vi "RT Driver VI.vi"(6 "Device Clock":string, 9 "Device Inputs FIFO":refnum<k33>, 10 "Device Outputs FIFO":refnum<k33>, 11 "Device Reference":T1 format="%.0x") -> ()   [LabVIEW 2019, in "Reset Hardware Engine.lvlib"]
uses:
  Reset Hardware Engine.lvlib
  <vilib>/NI VeriStand/Custom Device API/Custom Device Channel Type.ctl
  <vilib>/NI VeriStand/Custom Device API/Custom Device API.lvlib
  <vilib>/NI VeriStand/Custom Device Tools/Custom Device Utility Library/Custom Device Utility Library.lvlib
  <vilib>/NI VeriStand/Custom Device API/Message Response (String).ctl
  <vilib>/NI VeriStand/Custom Device API/Message Response (Byte Array).ctl
  Shared/Compiled.Settings.ctl
  Shared/Reset Hardware Shared.lvlib
  Shared/Constants.vi
  <vilib>/NI VeriStand/Custom Device API/Get Item Property (Variant).vi
  <vilib>/NI VeriStand/Custom Device API/Custom Device Item Ref.ctl
panel:
  in  "Initialization Status Notifier":refnum<notifier>
  in  "Status Notifier":refnum<notifier>
  # "Custom Device Template\nv1.0"
  # "Use this template as a starting point for creating a custom device code module. The input controls shown here are specially named controls that the system will use to provide the device loop with data. The controls are not required for the device loop to run. For instance, if the device doesn't produce any output data, then you don't need the Device Outputs FIFO control. If you do use these controls, however, they need to have these exact names to be functional."
  # "The optional status notifier element is used to notify the RT engine of the last state of the custom device, and to indicate the device has completed execution. If this control is not used, a default No Error value is returned to the system when the device finishes execution.\n\nNote: This error state is not checked until the system shuts down. Use an output status channel to send more immediate status values to the system."
  # "This optional input can be used to send the VeriStand Engine the final status of the custom device initalization process. If this control exists on the custom device front panel, the VeriStand Engine will wait for a status update before starting up. If the custom device reports an error, that will abort the execution of the current configuration in the VeriStand Engine.\n\nThis control can be deleted if the custom device does not need to send the initialization status update."
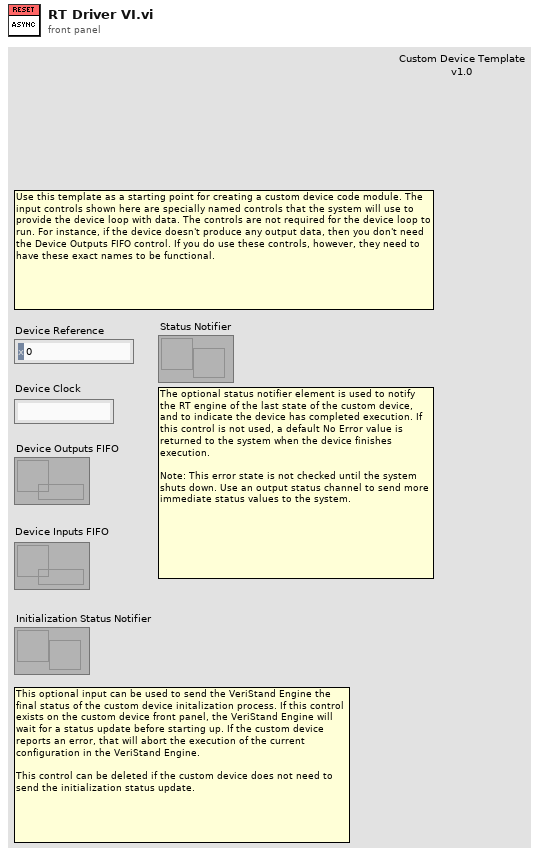
[diagram p1: front panel]
types:
  T1 = typedef "Custom Device API.lvlib/Custom Device Item Ref.ctl" = u64
  T2 = typedef "Reset Hardware Shared.lvlib/Compiled.Settings.ctl" = cluster{"Name":string, "Reset DAQmx AO":bool, "Reset XNET":bool}
  T3 = typedef "Custom Device API.lvlib/Custom Device Channel Type.ctl" = enum16{"Input", "Output"}
  T4 = typedef "Custom Device API.lvlib/Custom Device Engine Event Ref.ctl" = refnum<event-registration>
  T5 = typedef "Custom Device API.lvlib/Message Response (String).ctl" = cluster{"Response":string, "Error":errorcluster}
  T6 = typedef "Custom Device API.lvlib/Message Response (Byte Array).ctl" = cluster{"Response":u8[], "Error":errorcluster}
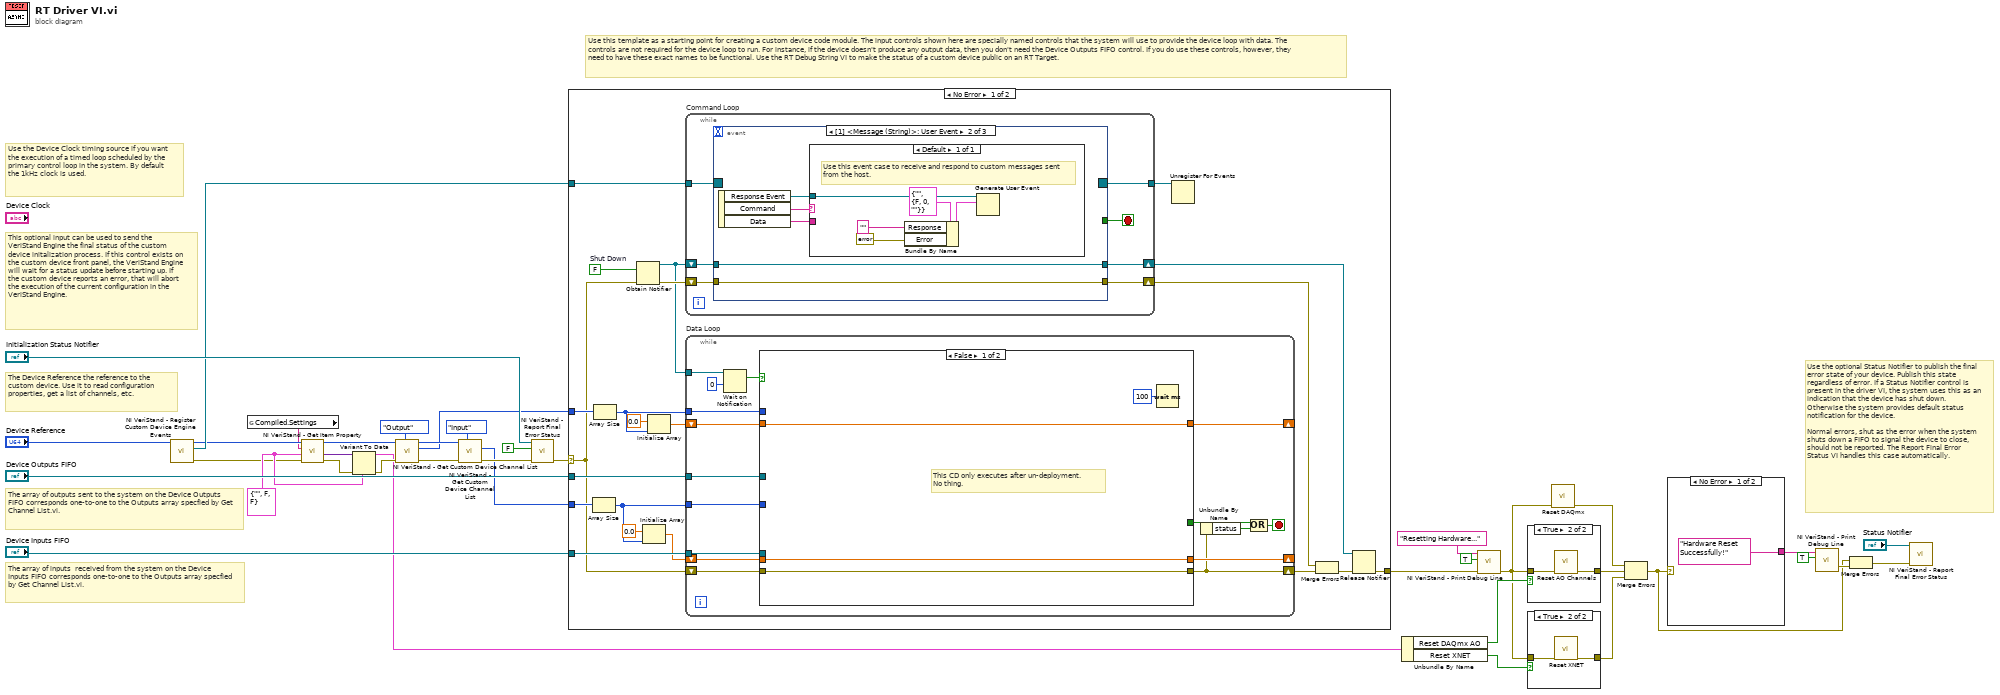
[diagram p0: block diagram]
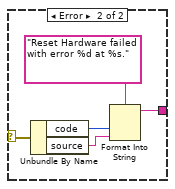
[diagram p4: hidden frame]
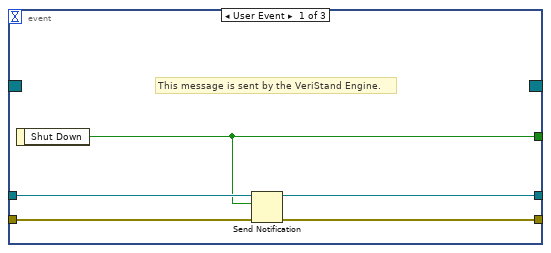
[diagram p5: hidden frame]
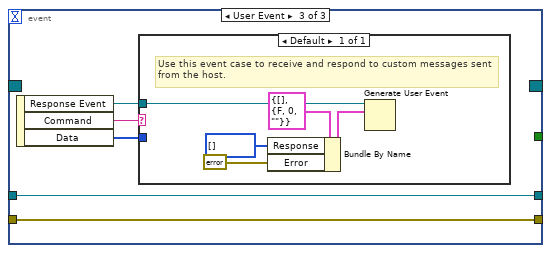
[diagram p6: hidden frame]
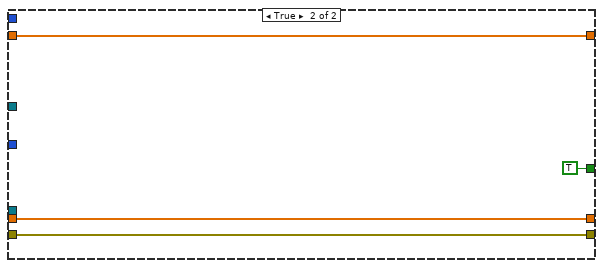
[diagram p7: hidden frame]
diagram:
  w17 = T2 {"Name"="", "Reset DAQmx AO"=FALSE, "Reset XNET"=FALSE} ("Compiled.Settings")
  # "This optional input can be used to send the VeriStand Engine the final status of the custom device initalization process. If this control exists on the custom device front panel, the VeriStand Engine will wait for a status update before starting up. If the custom device reports an error, that will abort the execution of the current configuration in the VeriStand Engine."
  # "The array of inputs  received from the system on the Device Inputs FIFO corresponds one-to-one to the Outputs array specfied by Get Channel List.vi."
  # "Use the optional Status Notifier to publish the final error state of your device. Publish this state regardless of error. If a Status Notifier control is present in the driver VI, the system uses this as an indication that the device has shut down. Otherwise the system provides default status notification for the device.\n\nNormal errors, shut as the error when the system shuts down a FIFO to signal the device to close, should not be reported. The Report Final Error Status VI handles this case automatically."
  # "The array of outputs sent to the system on the Device Outputs FIFO corresponds one-to-one to the Outputs array specfied by Get Channel List.vi."
  # "The Device Reference the reference to the custom device. Use it to read configuration properties, get a list of channels, etc."
  # "Use the Device Clock timing source if you want the execution of a timed loop scheduled by the primary control loop in the system. By default the 1kHz clock is used."
  # "Use this template as a starting point for creating a custom device code module. The input controls shown here are specially named controls that the system will use to provide the device loop with data. The controls are not required for the device loop to run. For instance, if the device doesn't produce any output data, then you don't need the Device Outputs FIFO control. If you do use these controls, however, they need to have these exact names to be functional. Use the RT Debug String VI to make the status of a custom device public on an RT Target."
  n1 = call <vilib>:"NI VeriStand - Register Custom Device Engine Events.vi"("Device Ref in"="Device Reference") -> ("error out"=w16:errorcluster, "Custom Device Engine Event Ref"=w27:T4, "Device Ref out"=w19:T1)  [unwired: 8 in]
  n2 = global read "Constants.vi" "Compiled.Settings"() -> (w7:string)
  n3 = call-poly <vilib>:"NI VeriStand - Get Item Property.vi"("error in (no error)"=w16, "Default Value"=w17, "Property Name"=w7, "Item Ref in"=w19) -> ("error out"=w20:errorcluster, "Value"=w21:variant, "Item Ref out"=w18:T1)  [unwired: 4 in, 1 out]
  n4 = Variant To Data(error in=w20, type=w17, Variant=w21) -> (data=w14:T2, error out=w15:errorcluster)
  n5 = call <vilib>:"NI VeriStand - Get Custom Device Channel List.vi"("Channel Type"=Custom_Device_Channel_Type."Output", "error in (no error)"=w15, "Device Ref in"=w18) -> ("error out"=w32:errorcluster, "Specified Channel Ref List"=w29:T1[], "Device Ref out"=w33:T1)  [unwired: 6 out]
  n6 = call <vilib>:"NI VeriStand - Get Custom Device Channel List.vi"("Channel Type"=Custom_Device_Channel_Type."Input", "error in (no error)"=w32, "Device Ref in"=w33) -> ("error out"=w38:errorcluster, "Specified Channel Ref List"=w30:T1[])  [unwired: 7 out]
  n7 = call <vilib>:"NI VeriStand - Report Final Error Status.vi"("error in (no error)"=w38, "Filter FIFO & Shutdown Errors (T)"=FALSE ("Filter FIFO Errors (T)"), "Status Notifier"="Initialization Status Notifier") -> ("error out"=w25:errorcluster)  [unwired: 8 out]
  n8 = case shown="No Error" w25 {
    selector: w25 -> [w41 w116]
    tunnel: "Device Outputs FIFO" -> [w58 _]
    tunnel: "Device Inputs FIFO" -> [w57 _]
    tunnel: w30 -> [w51 _]
    tunnel: w29 -> [w50 _]
    tunnel: w27 -> [w48 _]
    tunnel: [w46 w116] -> w23
    frame No Error {
      w47 = FALSE  # Shut Down
      n9 = Array Size(array=w51) -> (size(s)=w49:i32)
      n10 = Array Size(array=w50) -> (size(s)=w52:i32)
      n11 = Obtain Notifier(notification data type=w47, error in (no error)=w41) -> (notifier out=w44:refnum<notifier>, error out=w59:errorcluster)  [unwired: 2 in, 1 out]
      n12 = Initialize Array(0.0 ("element"), w49) -> (w53:dbl[])
      n13 = Initialize Array(0.0 ("element"), w52) -> (w54:dbl[])
      n14 = while "Command Loop" {
        tunnel: w48 -> [w66]
        tunnel: [w65] -> w45
        shift-right: [w62] -> w43
        shift-left: w44 -> [w63]
        shift-right: [w60] -> w39
        shift-left: w59 -> [w61]
        stop <- w64 stop-if-true
        n15 = event shown="[1] <Message (String)>: User Event" {
          selector: w66 -> [_ _ _]
          dyn-events: [_ _ _] -> w65
          timeout: _ -> [_ _ _]
          tunnel: [w69 _ _] -> w64
          tunnel: w63 -> [w70 w74 w84]
          tunnel: [w71 w74 w84] -> w62
          tunnel: w61 -> [w68 w72 w82]
          tunnel: [w67 w72 w82] -> w60
          event User Event {
            # "This message is sent by the VeriStand Engine."
            n16 = event-data() -> ("Shut Down"=w69:bool)  [unwired: 1 in]
            n17 = Send Notification(notification=w69, notifier=w70, error in (no error)=w68) -> (notifier out=w71:refnum<notifier>, error out=w67:errorcluster)
          }
          event User Event {
            n18 = event-data() -> ("Response Event"=w73:refnum<user-event>, "Command"=w76:string, "Data"=w75:string)  [unwired: 1 in]
            n19 = case shown="Default" w76 {
              tunnel: w75 -> [_]
              tunnel: w73 -> [w81]
              frame Default {
                # "Use this event case to receive and respond to custom messages sent from the host."
                n20 = Bundle By Name(cluster=T5 {"Response"="", "Error"={"status"=FALSE, "code"=0, "source"=""}} ("event data"), "Response"="", "Error"=errorcluster {"status"=FALSE, "code"=0, "source"=""}) -> (w79:T5)
                n21 = Generate User Event(user event=w81, event data cluster=w79) -> ()  [unwired: 2 in, 2 out]
              }
            }
          }
          event User Event {
            n22 = event-data() -> ("Response Event"=w83:refnum<user-event>, "Command"=w86:string, "Data"=w85:u8[])  [unwired: 1 in]
            n23 = case shown="Default" w86 {
              tunnel: w85 -> [_]
              tunnel: w83 -> [w91]
              frame Default {
                # "Use this event case to receive and respond to custom messages sent from the host."
                n24 = Bundle By Name(cluster=T6 {"Response"=[], "Error"={"status"=FALSE, "code"=0, "source"=""}} ("event data"), "Response"=u8[] [], "Error"=errorcluster {"status"=FALSE, "code"=0, "source"=""}) -> (w88:T6)
                n25 = Generate User Event(user event=w91, event data cluster=w88) -> ()  [unwired: 2 in, 2 out]
              }
            }
          }
        }
      }
      n26 = while "Data Loop" {
        shift-right: [w105] -> _
        shift-left: w53 -> [w106]
        shift-right: [w97] -> w42
        shift-left: w41 -> [w107]
        shift-right: [w103] -> _
        shift-left: w54 -> [w104]
        tunnel: w52 -> [w100]
        tunnel: w58 -> [w102]
        tunnel: w57 -> [w101]
        tunnel: w49 -> [w99]
        tunnel: w44 -> [w96]
        stop <- w92 stop-if-true
        n27 = Wait on Notification(notifier=w96, timeout in ms (-1)=0) -> (notification=w95:bool)  [unwired: 2 in, 3 out]
        n28 = case shown="False" w95 {
          tunnel: w107 -> [w109 w114]
          tunnel: w106 -> [w111 w115]
          tunnel: [w111 w115] -> w105
          tunnel: w104 -> [w110 w113]
          tunnel: [w110 w113] -> w103
          tunnel: w102 -> [_ _]
          tunnel: w101 -> [_ _]
          tunnel: w100 -> [_ _]
          tunnel: w99 -> [_ _]
          tunnel: [w109 w114] -> w97
          tunnel: [_ TRUE] -> w93
          frame False {
            # "This CD only executes after un-deployment.\nNo thing."
            n29 = Wait (ms)(milliseconds to wait=u32 100) -> ()  [unwired: 1 out]
          }
          frame True {
          }
        }
        n30 = Unbundle By Name(w97) -> ("status"=w94:bool)
        n31 = Compound Arithmetic op=OR(w93, w94) -> (w92:bool)
      }
      n32 = Unregister For Events(event registration refnum=w45) -> ()  [unwired: 1 in, 1 out]
      n33 = Merge Errors(w39, w42) -> (w40:errorcluster)
      n34 = Release Notifier(notifier=w43, error in (no error)=w40) -> (error out=w46:errorcluster)  [unwired: 1 in, 2 out]
    }
    frame Error {
    }
  }
  n35 = Unbundle By Name(w14) -> ("Reset DAQmx AO"=w11:bool, "Reset XNET"=w6:bool)
  n36 = call <vilib>:"NI VeriStand - Print Debug Line.vi"("error in (no error)"=w23, "Add to log file? (F)"=TRUE, "Message"="Resetting Hardware...") -> ("error out"=w3:errorcluster)  [unwired: 8 in]
  n37 = case shown="True" w11 {
    tunnel: w3 -> [w117 w119]
    tunnel: [w117 w118] -> w5
    frame False {
    }
    frame True {
      n38 = call "Reset AO Channels.vi"("error in (no error)"=w119) -> ("error out"=w118:errorcluster)  [unwired: 10 in]
    }
  }
  n39 = case shown="True" w6 {
    tunnel: w3 -> [w120 w122]
    tunnel: [w120 w121] -> w4
    frame False {
    }
    frame True {
      n40 = call "Reset XNET.vi"("error in (no error)"=w122) -> ("error out"=w121:errorcluster)  [unwired: 10 in]
    }
  }
  n41 = call "Reset DAQmx.vi"("error in (no error)"=w3) -> ("error out"=w2:errorcluster)  [unwired: 10 in]
  n42 = Merge Errors(w2, w5, w4) -> (w1:errorcluster)
  n43 = case shown="No Error" w1 {
    selector: w1 -> [_ w128]
    tunnel: ["Hardware Reset Successfully!" ("Message") w124] -> w8
    frame No Error {
    }
    frame Error {
      n44 = Unbundle By Name(w128) -> ("code"=w126:i32, "source"=w125:string)
      n45 = Format Into String(format string="Reset Hardware failed with error %d at %s.", w126, w125) -> (resulting string=w124:string)  [unwired: 2 in, 1 out]
    }
  }
  n46 = call <vilib>:"NI VeriStand - Print Debug Line.vi"("Add to log file? (F)"=TRUE, "Message"=w8) -> ("error out"=w10:errorcluster)  [unwired: 9 in]
  n47 = Merge Errors(w1, w10) -> (w9:errorcluster)
  n48 = call <vilib>:"NI VeriStand - Report Final Error Status.vi"("error in (no error)"=w9, "Status Notifier"="Status Notifier") -> ()  [unwired: 1 in, 9 out]
